vi "gaussian.vi"(0 "X":dbl[](array[numeric]), 1 "x0":dbl, 2 "sigma":dbl, 3 "bg":dbl, 4 "amplitude":dbl) -> (5 "Y":dbl[](array[numeric]))   [LabVIEW 2017]
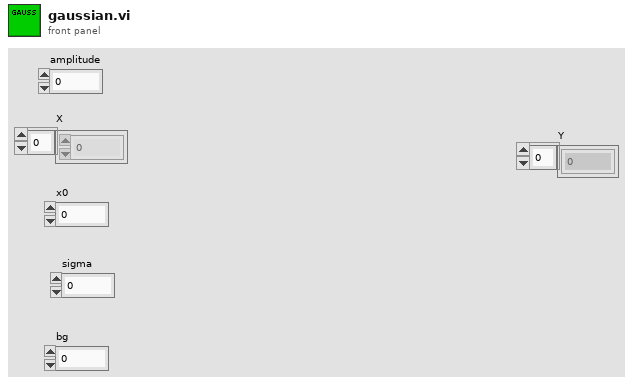
[diagram p1: front panel]
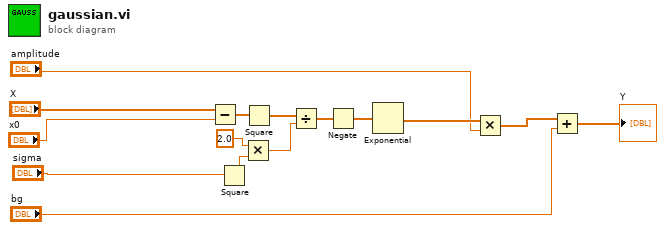
[diagram p0: block diagram]
diagram:
  n1 = Subtract(x="X", y="x0") -> (x-y=w13:dbl[])
  n2 = Square(x="sigma") -> (x^2=w9:dbl)
  n3 = Multiply(x=2.0, y=w9) -> (x*y=w8:dbl)
  n4 = Square(x=w13) -> (x^2=w12:dbl[])
  n5 = Divide(x=w12, y=w8) -> (x/y=w7:dbl[])
  n6 = Negate(x=w7) -> (-x=w6:dbl[])
  n7 = Exponential(1:w6) -> (0:w3:dbl[])
  n8 = Multiply(x=w3, y="amplitude") -> (x*y=w2:dbl[])
  n9 = Add(x=w2, y="bg") -> (x+y=→"Y":dbl[])
